vi "GA Get Backlash.vi"(7 "pCompDir":i32, 8 "error in (no error)":errorcluster caption="错误输入（无错误）", 9 "pCompChangeValue":dbl, 10 "pCompValue":i32, 11 "nAxisNum":i16) -> (0 "error out":errorcluster caption="错误输出", 1 "pCompChangeValue out":dbl, 2 "pCompValue out":i32, 3 "function return":i32, 5 "pCompDir out":i32)   [LabVIEW 2015, in "GAS.lvlib"]
doc: "extern \"C\" __declspec(dllimport) int GA_GetBacklash(short nAxisNum,long *pCompValue,double *pCompChangeValue,long *pCompDir);"
uses:
  <userlib>/BP_GAS/GAS.lvlib
  <userlib>/BP_GAS/GAS.dll
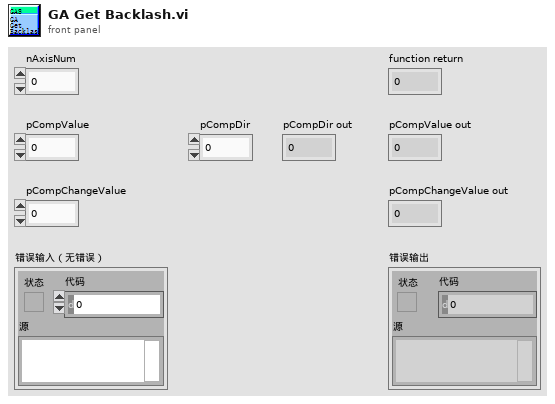
[diagram p1: front panel]
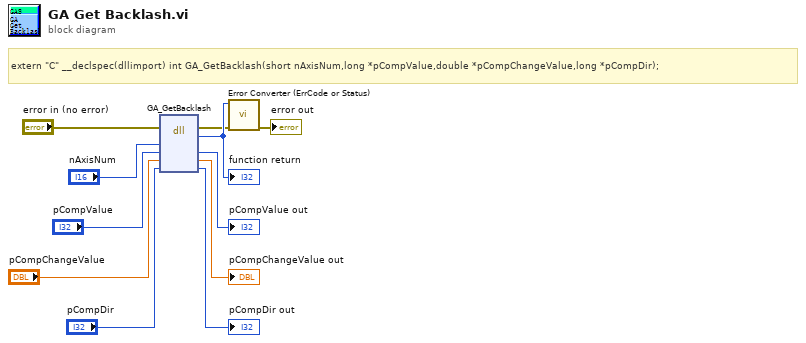
[diagram p0: block diagram]
diagram:
  # "extern \"C\" __declspec(dllimport) int GA_GetBacklash(short nAxisNum,long *pCompValue,double *pCompChangeValue,long *pCompDir);"
  n1 = dll-call lib="E:/Program Files (x86)/National Instruments/LabVIEW 2015/user.lib/BP_GAS/GAS.*" fn="GA_GetBacklash"(error in="error in (no error)", "nAxisNum"="nAxisNum", "pCompValue"="pCompValue", "pCompChangeValue"="pCompChangeValue", "pCompDir"="pCompDir") -> (error out=w2:errorcluster, w11:i32, "pCompValue"=→"pCompValue out":i32, "pCompChangeValue"=→"pCompChangeValue out":dbl, "pCompDir"=→"pCompDir out":i32)  [unwired: 3 in, 1 out]
  "function return" <- w11
  n2 = call "Error Converter (ErrCode or Status).vi"("error in (no error)"=w2, "error code"=w11) -> ("error out"=→"error out":errorcluster)  [unwired: 9 in]
